vi "Append a New Run.vi"(8 "error in (no error)":errorcluster, 9 "Style":refnum<class "Style.lvclass">, 10 "Text":string, 11 "xwpfParagraph in":refnum<class "xwpfParagraph.lvclass">) -> (0 "error out":errorcluster, 3 "xwpfParagraph out":refnum<class "xwpfParagraph.lvclass">)   [LabVIEW 2017, in "Word_Specific.lvlib" / "xwpfParagraph.lvclass"]
uses:
  xwpfParagraph.lvclass
  Styles/Style/Style.lvclass
  xwpfParagraph.lvclass/xwpfParagraph.ctl
  C:/Users/Neo/Desktop/Dev_Tools_BR/LabVIEW_NPOI/lib/NPOI 2.1.1/NPOI.OOXML.dll
  lib/NPOI 2.1.1/NPOI.OOXML.dll
  xwpfRun/xwpfRun.lvclass
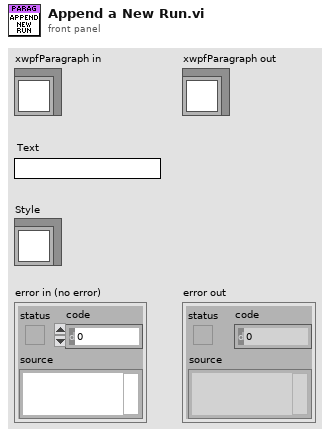
[diagram p1: front panel]
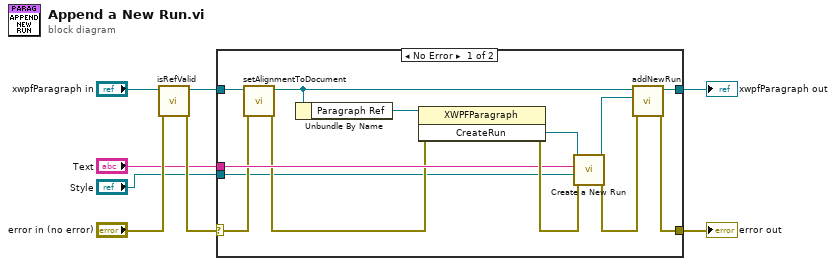
[diagram p0: block diagram]
diagram:
  n1 = call-dynamic "isRefValid.vi"("error in (no error)"="error in (no error)", "xwpfParagraph in"="xwpfParagraph in") -> ("error out"=w3:errorcluster, "xwpfParagraph out"=w5:refnum<class "xwpfParagraph.lvclass">)  [unwired: 8 in]
  n2 = case shown="No Error" w3 {
    selector: w3 -> [w11 w23]
    tunnel: [w13 w23] -> w8
    tunnel: [w16 w22] -> w6
    tunnel: w5 -> [w17 w22]
    tunnel: "Style" -> [w9 _]
    tunnel: "Text" -> [w18 _]
    frame No Error {
      n3 = call "setAlignmentToDocument.vi"("error in (no error)"=w11, "xwpfParagraph in"=w17) -> ("error out"=w10:errorcluster, "xwpfParagraph out"=w12:refnum<class "xwpfParagraph.lvclass">)  [unwired: 8 in]
      n4 = Unbundle By Name(w12) -> ("Paragraph Ref"=w21:refnum<k24>)
      n5 = invoke class="XWPFParagraph" method="CreateRun"(reference=w21, error in=w10) -> (error out=w19:errorcluster, "CreateRun"=w20:refnum<k24>)  [unwired: 1 in, 1 out]
      n6 = call "Create a New Run.vi"("error in (no error)"=w19, "Style"=w9, "Text"=w18, "Run Ref"=w20) -> ("error out"=w14:errorcluster, "xwpfRun out"=w15:refnum<class "xwpfRun.lvclass">)  [unwired: 6 in]
      n7 = call "addNewRun.vi"("error in (no error)"=w14, "New Run"=w15, "xwpfParagraph in"=w12) -> ("error out"=w13:errorcluster, "xwpfParagraph out"=w16:refnum<class "xwpfParagraph.lvclass">)  [unwired: 7 in]
    }
    frame Error {
    }
  }
  "error out" <- w8
  "xwpfParagraph out" <- w6
